vi "angle_to_setpoint.vi"() -> ()   [LabVIEW 2020]
uses:
  <vilib>/Math Plots/2D Math Plots/2D Compass/2D Compass XCtrl/2D Compass.xctl
  <vilib>/Math Plots/2D Math Plots/2D Compass/2D Compass Datatype/Public/Plot Helper (Vector).vi
  <vilib>/Math Plots/2D Math Plots/2D Compass/2D Compass Datatype/2D Compass Datatype.lvclass
panel:
  out "Theta":dbl
  out "Min":dbl
  out "Max":dbl
  out "2D Compass":refnum<class "2D Plot Datatype.lvclass">[](xcontrol)
  in  "Desired":dbl
  in  "Current":dbl
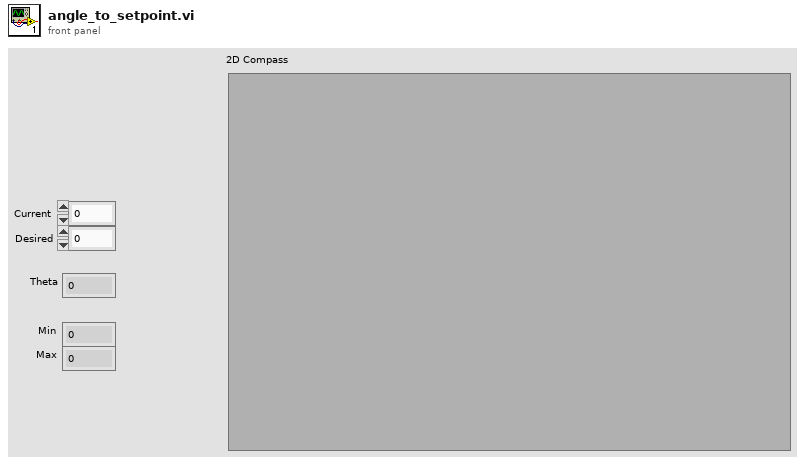
[diagram p1: front panel]
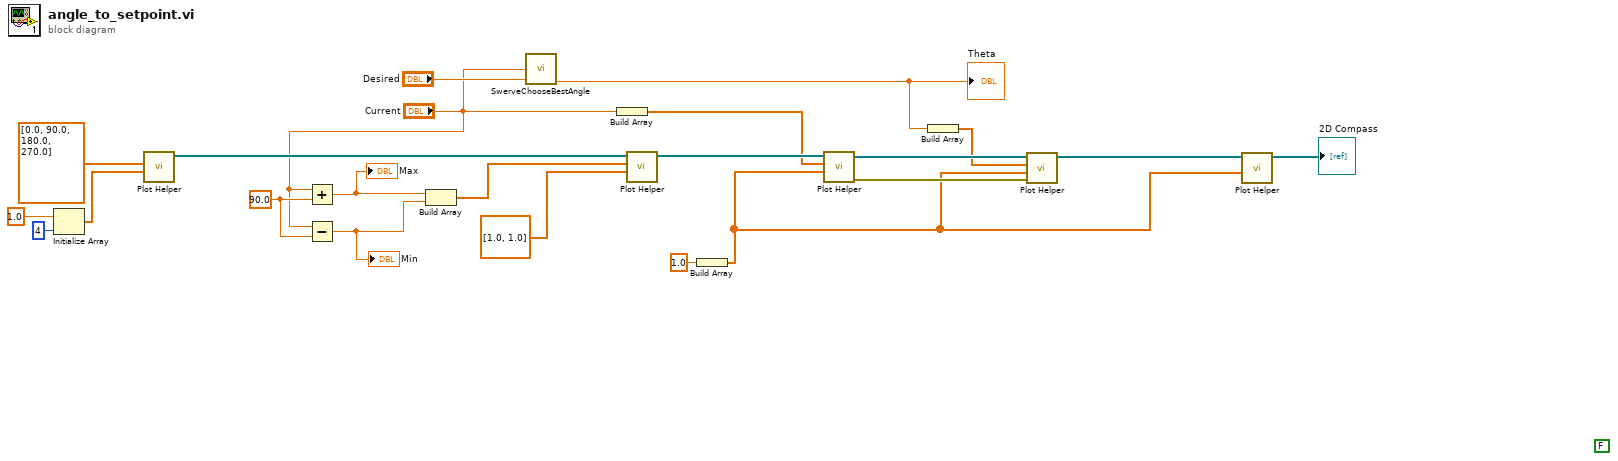
[diagram p0: block diagram]
diagram:
  (unwired) FALSE
  w12 = 90.0 ("y")
  n1 = Initialize Array(1.0 ("element"), 4 ("dimension size")) -> (w18:dbl[])
  n2 = call-poly <vilib>:"Plot Helper.vi"("radius vector"=w18, "theta vector"=dbl[] [0.0, 90.0, 180.0, 270.0]) -> ("2D Plot Class Obj Array out"=w19:refnum<class "2D Plot Datatype.lvclass">[])  [unwired: 2 in, 7 out]
  n3 = Add(x="Current", y=w12) -> (x+y=w6:dbl)
  "Max" <- w6
  n4 = Subtract(x="Current", y=w12) -> (x-y=w7:dbl)
  "Min" <- w7
  n5 = Build Array(w6, w7) -> (w13:dbl[])
  n6 = call "SwerveChooseBestAngle.vi"("Target Angle"="Desired", "Current Angle"="Current") -> ("Setpoint Angle"=w1:dbl)  [unwired: 5 in, 1 out]
  "Theta" <- w1
  n7 = Build Array("Current") -> (w15:dbl[])
  n8 = call-poly <vilib>:"Plot Helper.vi"("radius vector"=dbl[] [1.0, 1.0], "theta vector"=w13, "2D Plot Class Obj Array in"=w19) -> ("2D Plot Class Obj Array out"=w17:refnum<class "2D Plot Datatype.lvclass">[])  [unwired: 1 in, 7 out]
  n9 = Build Array(1.0 ("element")) -> (w4:dbl[])
  n10 = call-poly <vilib>:"Plot Helper.vi"("radius vector"=w4, "theta vector"=w15, "2D Plot Class Obj Array in"=w17) -> ("error out"=w10:errorcluster, "2D Plot Class Obj Array out"=w11:refnum<class "2D Plot Datatype.lvclass">[])  [unwired: 1 in, 6 out]
  n11 = Build Array(w1) -> (w5:dbl[])
  n12 = call-poly <vilib>:"Plot Helper.vi"("error in (no error)"=w10, "radius vector"=w4, "theta vector"=w5, "2D Plot Class Obj Array in"=w11) -> ("2D Plot Class Obj Array out"=w9:refnum<class "2D Plot Datatype.lvclass">[])  [unwired: 7 out]
  n13 = call-poly <vilib>:"Plot Helper.vi"("radius vector"=w4, "2D Plot Class Obj Array in"=w9) -> ("2D Plot Class Obj Array out"=→"2D Compass":refnum<class "2D Plot Datatype.lvclass">[])  [unwired: 2 in, 7 out]
